vi "Remove Item.vi"(8 "error in (no error)":errorcluster, 10 "Physical Channels":string, 11 "Parent Ref in":T1 format="%.0x") -> (0 "error out":errorcluster, 3 "Section Ref out":T1 format="%.0x")   [LabVIEW 2015]
uses:
  <vilib>/NI Veristand/Custom Device API/Custom Device Item Ref.ctl
  <vilib>/NI Veristand/Custom Device Tools/Custom Device Utility Library/NI VeriStand - Search for Item by Name.vi
  <vilib>/NI VeriStand/Custom Device Tools/Custom Device Utility Library/Custom Device Utility Library.lvlib
  <vilib>/NI VeriStand/Custom Device API/Custom Device API.lvlib
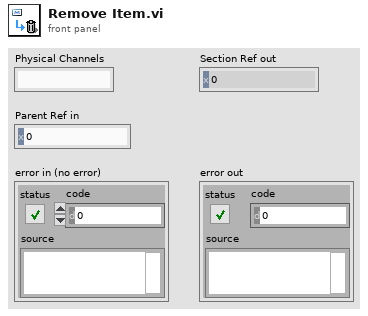
[diagram p1: front panel]
types:
  T1 = typedef "Custom Device API.lvlib/Custom Device Item Ref.ctl" = u64
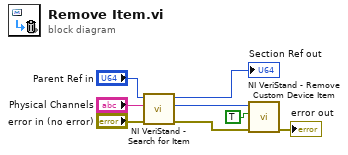
[diagram p0: block diagram]
diagram:
  n1 = call-poly <vilib>:"NI VeriStand - Search for Item.vi"("error in"="error in (no error)", "Item Name"="Physical Channels", "Section Ref in"="Parent Ref in") -> ("error out"=w3:errorcluster, "Item Ref"=w6:T1, "Section Ref out"=→"Section Ref out":T1)  [unwired: 5 in, 1 out]
  n2 = call <vilib>:"NI VeriStand - Remove Custom Device Item.vi"("error in (no error)"=w3, "Force Delete (F)"=TRUE, "Item Ref in"=w6) -> ("error out"=→"error out":errorcluster)  [unwired: 7 in, 1 out]
